vi "Test Read Timeout.vi"(8 "error in (no error)":errorcluster, 11 "TestCase in":refnum<class "Test WebSockets Core.lvclass">) -> (0 "error out":errorcluster, 3 "TestCase out":refnum<class "Test WebSockets Core.lvclass">)   [LabVIEW 2013, in "Test WebSockets Core.lvclass"]
uses:
  Test WebSockets Core.lvclass
  WebSockets/WebSocket Client/WebSocket Client.lvclass
  <vilib>/addons/_JKI Toolkits/VI Tester/TestCase.llb/TestCase.lvclass
  WebSockets/WebSocket/WebSocket.lvclass
  Sockets/VISA TCP Socket/VISA TCP.lvclass
panel:
  out "Data":string
  out "Read time":u32
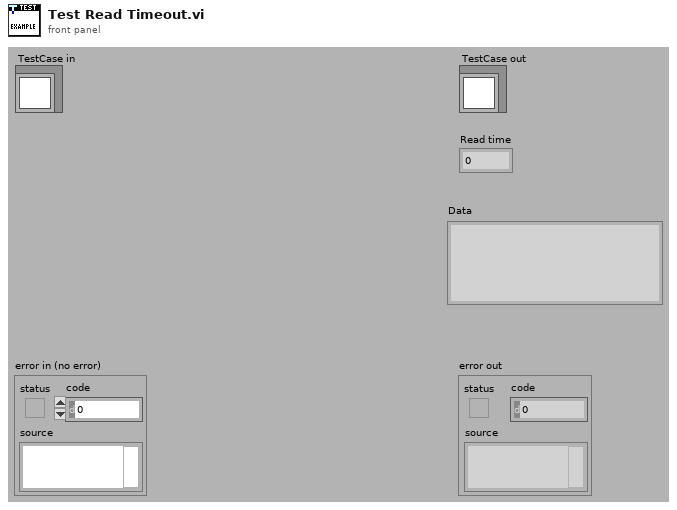
[diagram p1: front panel]
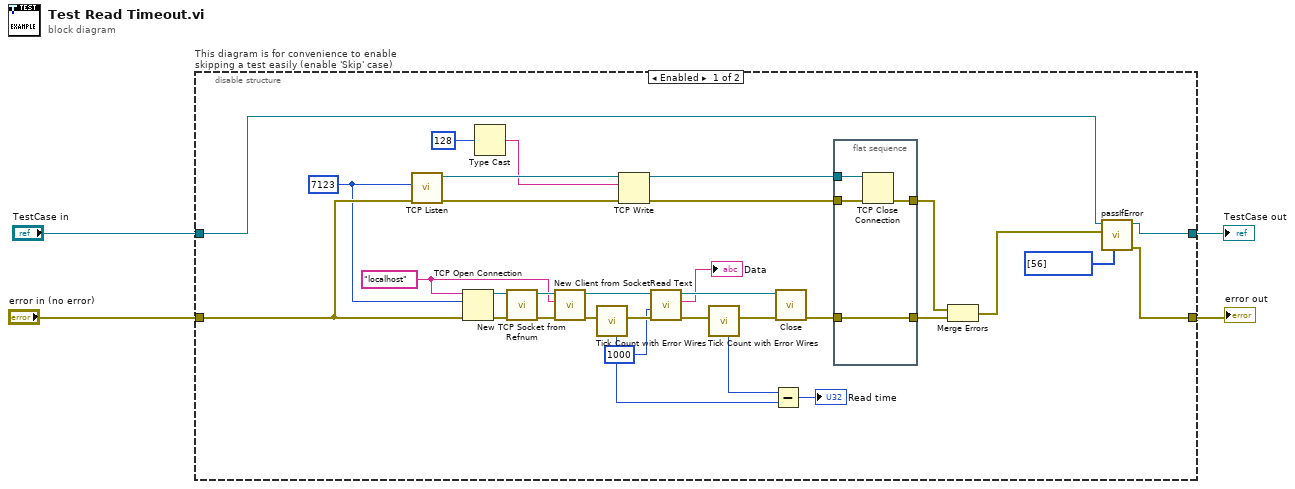
[diagram p0: block diagram]
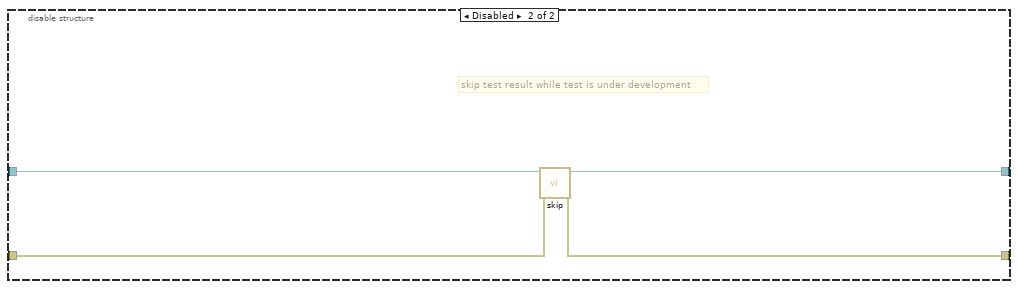
[diagram p2: hidden frame]
diagram:
  n1 = disable-structure "This diagram is for convenience to enable skipping a test easily (enable 'Skip' case)" shown="Enabled" {
    disable-tunnel: "TestCase in" -> [w8 w44]
    disable-tunnel: [w9 w42] -> w1
    disable-tunnel: [w5 w43] -> w3
    disable-tunnel: "error in (no error)" -> [w36 w41]
    frame Enabled {
      w14 = "localhost" ("address")
      w35 = u16 7123 ("port")
      n2 = call <vilib>:"TCP Listen.vi"("error in (no error)"=w36, "port"=w35) -> ("error out"=w34:errorcluster, "connection ID"=w33:refnum<k5>)  [unwired: 5 in, 3 out]
      n3 = TCP Open Connection(address=w14, remote port or service name=w35, error in (no error)=w36) -> (connection ID=w12:refnum<k5>, error out=w13:errorcluster)  [unwired: 2 in]
      n4 = Type Cast(x=u8 128) -> (*(type *) &x=w31:string)  [unwired: 1 in]
      n5 = call "New TCP Socket from Refnum.vi"("error in (no error)"=w13, "TCP Network Connection Refnum"=w12) -> ("error out"=w16:errorcluster, "VISA TCP out"=w15:refnum<class "VISA TCP.lvclass">)  [unwired: 8 in]
      n6 = call "New Client from Socket.vi"("error in (no error)"=w16, "WebSocket URL"=w14, "Socket in"=w15) -> ("error out"=w11:errorcluster, "WebSocket Client out"=w10:refnum<class "WebSocket Client.lvclass">)  [unwired: 7 in]
      n7 = call "Tick Count with Error Wires.vi"("error in (no error)"=w11) -> ("error out"=w22:errorcluster, "millisecond timer value"=w20:u32)  [unwired: 9 in]
      n8 = TCP Write(connection ID=w33, data in=w31, error in (no error)=w34) -> (connection ID out=w25:refnum<k5>, error out=w26:errorcluster)  [unwired: 1 in, 1 out]
      n9 = call-dynamic "Read Text.vi"("error in (no error)"=w22, "timeout ms (5000)"=1000, "WebSocket in"=w10) -> ("error out"=w30:errorcluster, "Data"=→"Data":string, "WebSocket out"=w24:refnum<class "WebSocket Client.lvclass">)  [unwired: 6 in]
      n10 = call "Tick Count with Error Wires.vi"("error in (no error)"=w30) -> ("error out"=w23:errorcluster, "millisecond timer value"=w21:u32)  [unwired: 9 in]
      n11 = Subtract(x=w21, y=w20) -> (x-y=→"Read time":u32)
      n12 = call-dynamic "Close.vi"("error in (no error)"=w23, "WebSocket in"=w24) -> ("error out"=w29:errorcluster)  [unwired: 9 in]
      n13 = flat-sequence {
        tunnel: w29 -> [w40]
        tunnel: [w40] -> w28
        tunnel: [w39] -> w27
        tunnel: w26 -> [w38]
        tunnel: w25 -> [w37]
        frame #0 {
          n14 = TCP Close Connection(connection ID=w37, error in (no error)=w38) -> (error out=w39:errorcluster)  [unwired: 1 in, 1 out]
        }
      }
      n15 = Merge Errors(w27, w28) -> (w6:errorcluster)
      n16 = call-dynamic "passIfError.vi"("passing error codes (default = any error code)"=i32[] [56], "error"=w6, "TestCase in"=w8) -> ("error out"=w5:errorcluster, "TestCase out"=w9:refnum<class "Test WebSockets Core.lvclass">)  [unwired: 7 in]
    }
    frame Disabled {
      # "skip test result while test is under development"
      n17 = call <vilib>:"skip.vi"("error in (no error)"=w41, "TestCase in"=w44) -> ("error out"=w43:errorcluster, "TestCase out"=w42:refnum<class "Test WebSockets Core.lvclass">)  [unwired: 8 in]
    }
  }
  "error out" <- w3
  "TestCase out" <- w1
